vi "SD Module_UI.vi"(8 "error in (no error)":errorcluster, 11 "Node Ptr":T16 format="%.0x") -> (0 "error out":errorcluster)   [LabVIEW 2017, in "Modules.lvlib" / "SD Module.lvclass"]
uses:
  SD Module.lvclass
  Type Defs/_nicrio_TimebaseControl.ctl
  Type Defs/_nicrio_IndexModeControl.ctl
  Type Defs/_nicrio_PeriodControl.ctl
  Type Defs/_nicrio_DriveChanFromCounterControl.ctl
  Type Defs/_nicrio_TerminalCountOutputModeControl.ctl
  Type Defs/_nicrio_GateSourceControl.ctl
  Type Defs/_nicrio_CountEventControl.ctl
  Type Defs/_nicrio_TerminalCountControl.ctl
  Type Defs/_nicrio_CountSourceControl.ctl
  Type Defs/_nicrio_MeasurementModeControl.ctl
  Type Defs/_nicrio_CountDownControl.ctl
  <vilib>/NI Veristand/Custom Device API/Custom Device Item Ref.ctl
  RSI Module/SubPanel Command.ctl
  Type Defs/_nicrio_SpecialtyModeControl.ctl
  Type Defs/_nicrio_InputFilterControl.ctl
  Type Defs/_nicrio_ChannelsControl.ctl
  Type Defs/Quadrature Control Refs.ctl
  Type Defs/Counter Control Refs.ctl
  Type Defs/Main Control Refs.ctl
  Type Defs/SD Control Refs.ctl
  Type Defs/CDO Control Refs.ctl
  Type Defs/PWM Control Refs.ctl
  RSI Module/Slot Settings.ctl
  RSI Module/Module Models.ctl
  C:/Users/dbuck/Documents/GitHub/Scan-Engine-Custom-Device-Classes/Source/RSI Module/RSI Module.lvclass
  SD Module.lvclass/SD Module.ctl
  RSI Module/Debug.vi
  RSI Module/RSI Module.lvclass
  <resource>/objmgr/cRIO.rc
  Modules.lvlib
  <vilib>/NI Veristand/Custom Device API/Custom Device API.lvlib
panel:
  in  "Channels":T1
  in  "Input Filter":T2=128 items=["1 us"=0, "16 us"=1, "256 us"=2, "4096 us"=3, "Disabled"=128]
  in  "SD Tabs":T3(tab)
  in  "Measurement Type":T4 items=["High Pulse"=3, "Low Pulse"=4, "Most Recent"=5]
  in  "Measurement Edge":T4 items=["Rising Edge", "Falling Edge"]
  in  "Output Mode":T5 caption="Terminal Count Output Mode" items=["Toggle, Reset Off", "Toggle, Reset On", "On Pulse", "Off Pulse"]
  in  "Gate Mode":T6 items=["Always Enabled"=3, "Next Channel"=1]
  in  "Counter Event":T4 items=["Rising Edge", "Falling Edge", "Any Edge"]
  in  "Terminal Count":T7=4294967296 min=1 max=4294967296
  in  "Counter Source":T8 items=["This Channel", "Terminal Count of Previous Channel"]
  in  "Frequency Timebase":T9 items=["256 us", "512 us", "1024 us", "2048 us", "4096 us", "8192 us", "16384 us", "32768 us"]
  in  "Measurement Mode":T10 items=["Count Edges", "Period Measurement", "Pulse Width Measurement", "Frequency Measurement"]
  in  "Count Direction":T11 items=["Count Up", "Count Down"]
  in  "Channel Mode":T12 caption="Counter Driven" items=["Disabled", "Enabled"]
  in  "Drive From Slot":u16(ring) items=["Slot 1", "Slot 2", "Slot 3", "Slot 4", "Slot 5", "Slot 6", "Slot 7", "Slot 8"]
  in  "Frequency (Period)":T13=4 items=["1 Hz (1,000,000 us)", "50 Hz (20,000 us)", "250 Hz (4,000 us)", "500 Hz (2,000 us)", "1 kHz (1,000 us)", "5 kHz (200 us)", "10 kHz (100 us)", "20 kHz (50 us)"]
  in  "Velocity Timebase":T9 items=["256 us", "512 us", "1024 us", "2048 us", "4096 us", "8192 us", "16384 us", "32768 us"]
  in  "Index Mode":T14 items=["Disabled", "Phase B0 A0", "Phase B0 A1", "Phase B1 A0", "Phase B1 A1"]
  in  "Specialty Mode":T15 items=["None", "Counter", "Counter-Driven Output", "Pulse-Width Modulation", "Quadrature"]
  in  "SubPanel Event":refnum<user-event>
  in  "Header":cluster{"Section Name":string}={"Section Name"="NI 9205 Settings"}
  # "When in quadrature mode, the A, B, and index channels are the first, second, and third input lines respectively. Modules with six or more digital inputs use successive blocks of three channels to instantiate additional quadratures in the same pattern."
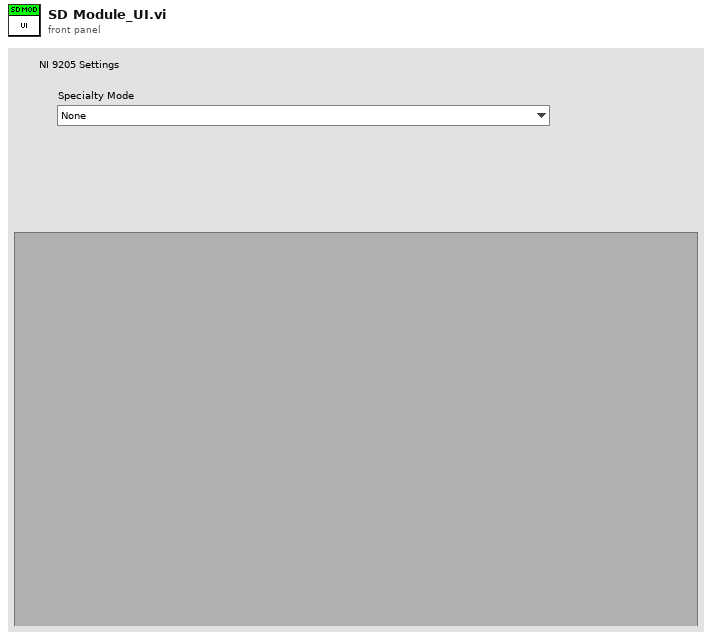
[diagram p1: front panel]
types:
  T1 = typedef "Modules.lvlib/SD Module.lvclass/_nicrio_ChannelsControl.ctl" = i32
  T2 = typedef "Modules.lvlib/SD Module.lvclass/_nicrio_InputFilterControl.ctl" = u16
  T3 = enum32{"Normal", "Counter", "Counter Output", "PWM", "Quadrature", "Error"}
  T4 = typedef "Modules.lvlib/SD Module.lvclass/_nicrio_CountEventControl.ctl" = u16
  T5 = typedef "Modules.lvlib/SD Module.lvclass/_nicrio_TerminalCountOutputModeControl.ctl" = u16
  T6 = typedef "Modules.lvlib/SD Module.lvclass/_nicrio_GateSourceControl.ctl" = u16
  T7 = typedef "Modules.lvlib/SD Module.lvclass/_nicrio_TerminalCountControl.ctl" = u64
  T8 = typedef "Modules.lvlib/SD Module.lvclass/_nicrio_CountSourceControl.ctl" = u16
  T9 = typedef "Modules.lvlib/SD Module.lvclass/_nicrio_TimebaseControl.ctl" = u16
  T10 = typedef "Modules.lvlib/SD Module.lvclass/_nicrio_MeasurementModeControl.ctl" = u16
  T11 = typedef "Modules.lvlib/SD Module.lvclass/_nicrio_CountDownControl.ctl" = u16
  T12 = typedef "Modules.lvlib/SD Module.lvclass/_nicrio_DriveChanFromCounterControl.ctl" = u16
  T13 = typedef "Modules.lvlib/SD Module.lvclass/_nicrio_PeriodControl.ctl" = u16
  T14 = typedef "Modules.lvlib/SD Module.lvclass/_nicrio_IndexModeControl.ctl" = u16
  T15 = typedef "Modules.lvlib/SD Module.lvclass/_nicrio_SpecialtyModeControl.ctl" = u16
  T16 = typedef "Custom Device API.lvlib/Custom Device Item Ref.ctl" = u64
  T17 = typedef "Modules.lvlib/SD Module.lvclass/PWM Control Refs.ctl" = cluster{"Frequency (Period)":refnum<vi>}
  T18 = typedef "Modules.lvlib/SD Module.lvclass/CDO Control Refs.ctl" = cluster{"Drive From Slot":refnum<vi>, "Channel Mode":refnum<vi>}
  T19 = typedef "Modules.lvlib/SD Module.lvclass/SD Control Refs.ctl" = cluster{"Main Control Refs":T20, "Counter Control Refs":T21, "CDO Control Refs":T18, "PWM Control Refs":T17, "Quadrature Control Refs":T22}
  T20 = typedef "Modules.lvlib/SD Module.lvclass/Main Control Refs.ctl" = cluster{"Specialty Mode":refnum<vi>, "Input Filter":refnum<vi>, "SD Tabs":refnum<vi>, "Channels":refnum<vi>, "Non-SD Subpanel":refnum<vi>}
  T21 = typedef "Modules.lvlib/SD Module.lvclass/Counter Control Refs.ctl" = cluster{"Measurement Mode":refnum<vi>, "Counter Event":refnum<vi>, "Counter Source":refnum<vi>, "Count Direction":refnum<vi>, "Terminal Count":refnum<vi>, "Output Mode":refnum<vi>, "Gate Mode":refnum<vi>, "Measurement Edge":refnum<vi>, "Measurement Type":refnum<vi>, "Frequency Timebase":refnum<vi>}
  T22 = typedef "Modules.lvlib/SD Module.lvclass/Quadrature Control Refs.ctl" = cluster{"Velocity Timebase":refnum<vi>, "Index Mode":refnum<vi>}
  T23 = typedef "Modules.lvlib/RSI Module.lvclass/Module Models.ctl" = enum16{"Empty", "NI 9201", "NI 9203", "NI 9205", "NI 9206", "NI 9207", "NI 9208", "NI 9211", "NI 9212", "NI 9213", "NI 9214", "NI 9215", "NI 9217", "NI 9219", "NI 9220", "NI 9221", "NI 9222", "NI 9223", "NI 9225", "NI 9227", "NI 9229", "NI 9233", "NI 9234", "NI 9235", "NI 9236", "NI 9237", "NI 9239", "NI 9242", "NI 9244", "NI 9263", "NI 9264", "NI 9265", "NI 9269", "NI 9375", "NI 9401", "NI 9402", "NI 9403", "NI 9411", "NI 9421", "NI 9422", "NI 9423", "NI 9425", "NI 9426", "NI 9435", "NI 9437", "NI 9472", "NI 9474", "NI 9475", "NI 9476", "NI 9477", "NI 9478", "NI 9481", "NI 9482", "NI 9485"}
  T24 = typedef "Modules.lvlib/RSI Module.lvclass/Slot Settings.ctl" = cluster{"Slot":u32, "EtherCAT?":bool}
  T25 = typedef "Modules.lvlib/RSI Module.lvclass/SubPanel Command.ctl" = enum16{"Stop"}
  T26 = typedef "Modules.lvlib/SD Module.lvclass/CDO Channel.ctl" = cluster{"Counter driven enabled":bool}
  T27 = typedef "Modules.lvlib/SD Module.lvclass/Quadrature Channel.ctl" = cluster{"Timebase":u32, "Index Mode":u32}
  T28 = typedef "Modules.lvlib/SD Module.lvclass/Counter Channel.ctl" = cluster{"Measurement Mode":u32, "Count Edges":T29, "Period Measurement":T30, "Pulse Width Measurement":T31, "Frequency Measurement":T32}
  T29 = typedef "Modules.lvlib/SD Module.lvclass/Count Edges.ctl" = cluster{"Counter Event":u32, "Counter Source":u32, "Counter Direction":u32, "Terminal Count":u32, "Output Mode":u32, "Gate Mode":u32}
  T30 = typedef "Modules.lvlib/SD Module.lvclass/Period Measurement.ctl" = cluster{"Measurement Edge":u32}
  T31 = typedef "Modules.lvlib/SD Module.lvclass/Pulse Width Measurement.ctl" = cluster{"Measurement Type":u32}
  T32 = typedef "Modules.lvlib/SD Module.lvclass/Frequency Measurement.ctl" = cluster{"Measurement Edge":u32, "Measurement Timebase":u32}
  T33 = typedef "Modules.lvlib/SD Module.lvclass/PWM Channel.ctl" = cluster{"PWM frequency":u32}
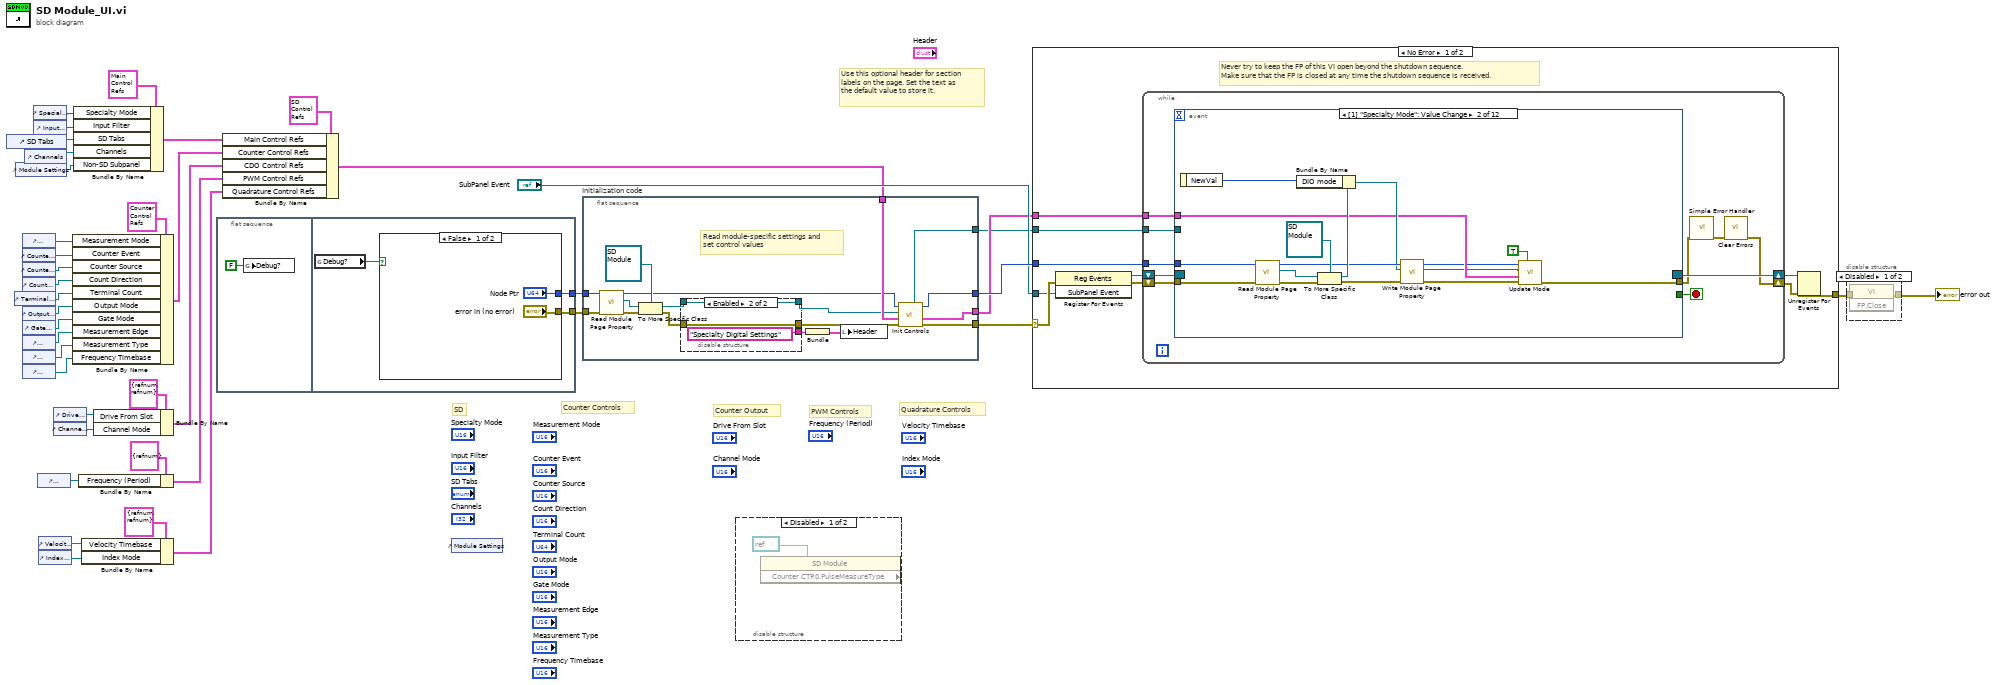
[diagram p0: block diagram]
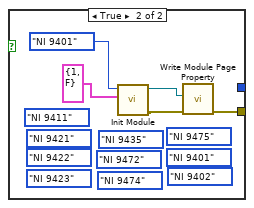
[diagram p3: hidden frame]
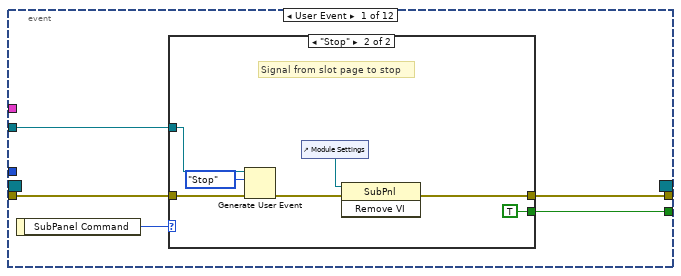
[diagram p4: hidden frame]
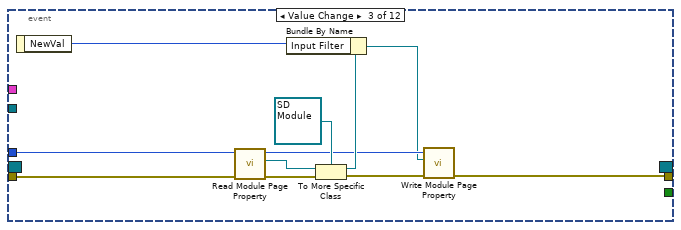
[diagram p6: hidden frame]
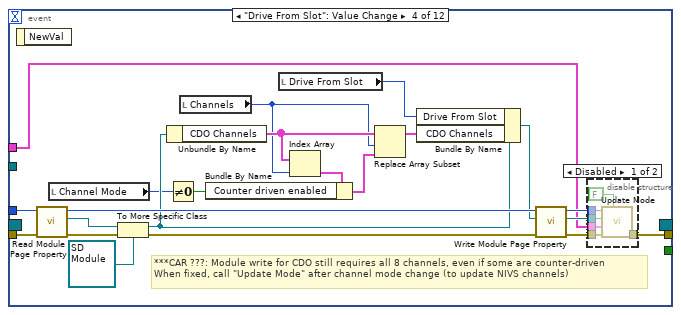
[diagram p7: hidden frame]
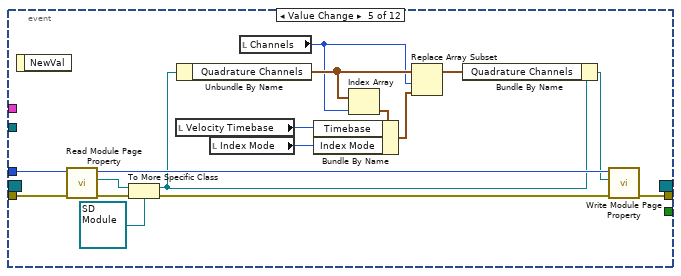
[diagram p9: hidden frame]
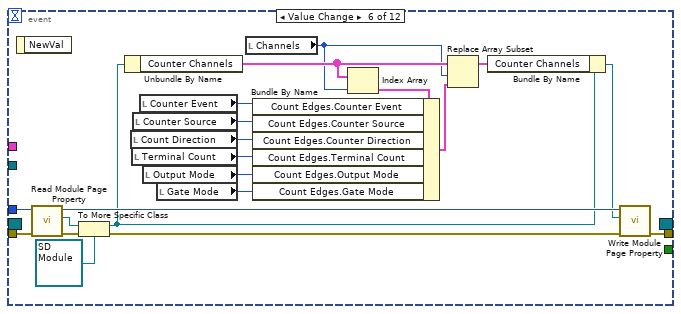
[diagram p10: hidden frame]
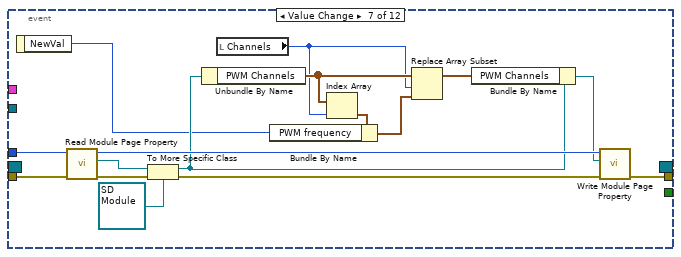
[diagram p11: hidden frame]
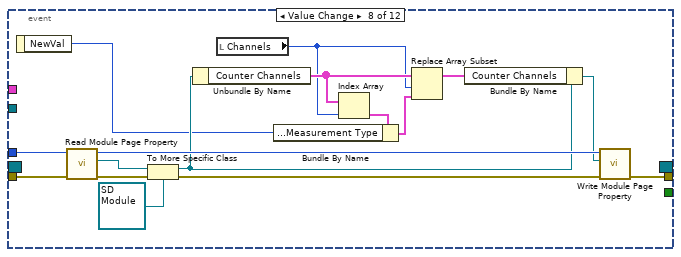
[diagram p12: hidden frame]
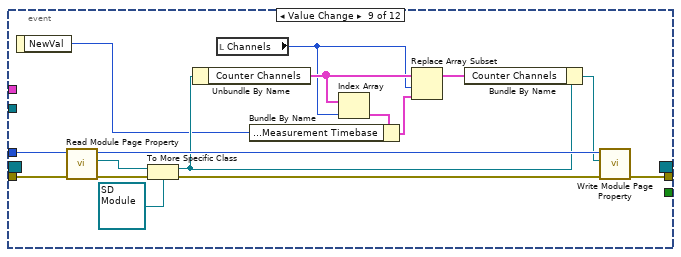
[diagram p13: hidden frame]
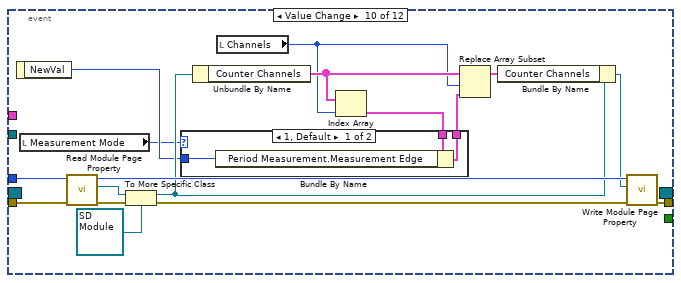
[diagram p14: hidden frame]
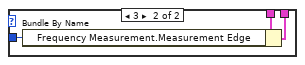
[diagram p15: hidden frame]
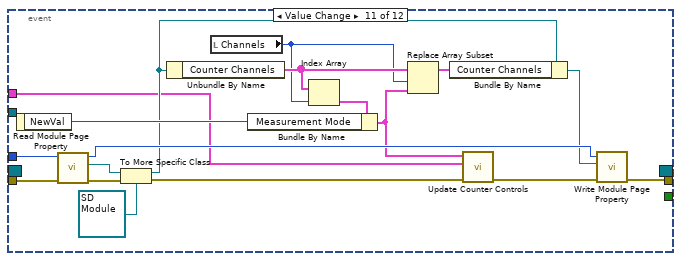
[diagram p16: hidden frame]
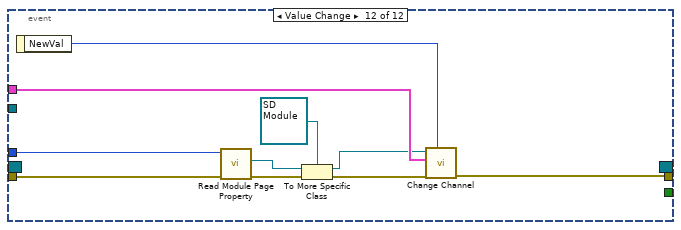
[diagram p17: hidden frame]
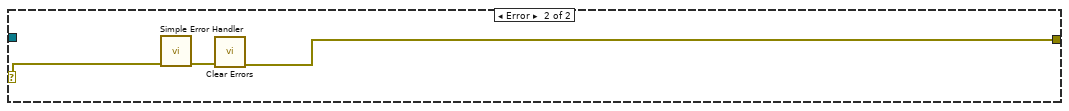
[diagram p18: hidden frame]
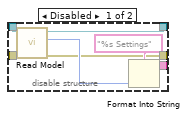
[diagram p19: hidden frame]
diagram:
  # "Counter Output"
  # "Quadrature Controls"
  # "Counter Controls"
  # "PWM Controls"
  # "SD"
  # "Use this optional header for section labels on the page. Set the text as the default value to store it."
  n1 = control-ref of="SD Tabs"() -> (w16:refnum<vi>)
  n2 = control-ref of="Terminal Count"() -> (w25:refnum<vi>)
  n3 = control-ref of="Module Settings"() -> (w2:refnum<vi>)
  n4 = control-ref of="Measurement Mode"() -> (w29:refnum<vi>)
  n5 = control-ref of="Counter Event"() -> (w28:refnum<vi>)
  n6 = control-ref of="Counter Source"() -> (w27:refnum<vi>)
  n7 = control-ref of="Count Direction"() -> (w26:refnum<vi>)
  n8 = control-ref of="Output Mode"() -> (w24:refnum<vi>)
  n9 = control-ref of="Gate Mode"() -> (w23:refnum<vi>)
  n10 = control-ref of="Measurement Edge"() -> (w22:refnum<vi>)
  n11 = control-ref of="Measurement Type"() -> (w21:refnum<vi>)
  n12 = control-ref of="Frequency Timebase"() -> (w20:refnum<vi>)
  n13 = control-ref of="Channels"() -> (w15:refnum<vi>)
  n14 = control-ref of="Specialty Mode"() -> (w18:refnum<vi>)
  n15 = control-ref of="Input Filter"() -> (w17:refnum<vi>)
  n16 = control-ref of="Frequency (Period)"() -> (w10:refnum<vi>)
  n17 = control-ref of="Velocity Timebase"() -> (w40:refnum<vi>)
  n18 = control-ref of="Index Mode"() -> (w39:refnum<vi>)
  n19 = control-ref of="Drive From Slot"() -> (w13:refnum<vi>)
  n20 = control-ref of="Channel Mode"() -> (w12:refnum<vi>)
  n21 = Bundle By Name(cluster=T21 {"Measurement Mode"=refnum, "Counter Event"=refnum, "Counter Source"=refnum, "Count Direction"=refnum, "Terminal Count"=refnum, "Output Mode"=refnum, "Gate Mode"=refnum, "Measurement Edge"=refnum, "Measurement Type"=refnum, "Frequency Timebase"=refnum} ("Counter Control Refs"), "Measurement Mode"=w29, "Counter Event"=w28, "Counter Source"=w27, "Count Direction"=w26, "Terminal Count"=w25, "Output Mode"=w24, "Gate Mode"=w23, "Measurement Edge"=w22, "Measurement Type"=w21, "Frequency Timebase"=w20) -> (w7:T21)
  n22 = Bundle By Name(cluster=T20 {"Specialty Mode"=refnum, "Input Filter"=refnum, "SD Tabs"=refnum, "Channels"=refnum, "Non-SD Subpanel"=refnum} ("Main Control Refs"), "Specialty Mode"=w18, "Input Filter"=w17, "SD Tabs"=w16, "Channels"=w15, "Non-SD Subpanel"=w2) -> (w8:T20)
  n23 = Bundle By Name(cluster=T17 {"Frequency (Period)"=refnum} ("PWM Control Refs"), "Frequency (Period)"=w10) -> (w5:T17)
  n24 = Bundle By Name(cluster=T22 {"Velocity Timebase"=refnum, "Index Mode"=refnum} ("Quadrature Control Refs"), "Velocity Timebase"=w40, "Index Mode"=w39) -> (w38:T22)
  n25 = Bundle By Name(cluster=T18 {"Drive From Slot"=refnum, "Channel Mode"=refnum} ("CDO Control Refs"), "Drive From Slot"=w13, "Channel Mode"=w12) -> (w6:T18)
  n26 = flat-sequence {
    tunnel: [w45] -> w36
    tunnel: [w44] -> w35
    frame #0 {
      n27 = global write "Debug.vi" "Debug?"(FALSE ("Debug?")) -> ()
    }
    frame #1 {
      n28 = global read "Debug.vi" "Debug?"() -> (w43:bool)
      n29 = case shown="False" w43 {
        tunnel: ["Node Ptr" _] -> w45
        tunnel: ["error in (no error)" w52] -> w44
        frame False {
        }
        frame True {
          (unwired) Module_Models."NI 9402" ("Module Model")
          (unwired) Module_Models."NI 9401" ("Module Model")
          (unwired) Module_Models."NI 9411" ("Module Model")
          (unwired) Module_Models."NI 9475" ("Module Model")
          (unwired) Module_Models."NI 9474" ("Module Model")
          (unwired) Module_Models."NI 9472" ("Module Model")
          (unwired) Module_Models."NI 9435" ("Module Model")
          (unwired) Module_Models."NI 9423" ("Module Model")
          (unwired) Module_Models."NI 9422" ("Module Model")
          (unwired) Module_Models."NI 9421" ("Module Model")
          n30 = call "Init Module.vi"("Slot Settings"=T24 {"Slot"=1, "EtherCAT?"=FALSE}, "Module Model"=Module_Models."NI 9401") -> ("error out"=w49:errorcluster, "RSI Module out"=w48:refnum<class "RSI Module.lvclass">)  [unwired: 8 in]
          n31 = call "Write Module Page Property.vi"("error in (no error)"=w49, "RSI Module"=w48) -> ("error out"=w52:errorcluster)  [unwired: 7 in, 2 out]
        }
      }
    }
  }
  n32 = Bundle By Name(cluster=T19 {"Main Control Refs"={"Specialty Mode"=refnum, "Input Filter"=refnum, "SD Tabs"=refnum, "Channels"=refnum, "Non-SD Subpanel"=refnum}, "Counter Control Refs"={"Measurement Mode"=refnum, "Counter Event"=refnum, "Counter Source"=refnum, "Count Direction"=refnum, "Terminal Count"=refnum, "Output Mode"=refnum, "Gate Mode"=refnum, "Measurement Edge"=refnum, "Measurement Type"=refnum, "Frequency Timebase"=refnum}, "CDO Control Refs"={"Drive From Slot"=refnum, "Channel Mode"=refnum}, "PWM Control Refs"={"Frequency (Period)"=refnum}, "Quadrature Control Refs"={"Velocity Timebase"=refnum, "Index Mode"=refnum}} ("SD Control Refs"), "Main Control Refs"=w8, "Counter Control Refs"=w7, "CDO Control Refs"=w6, "PWM Control Refs"=w5, "Quadrature Control Refs"=w38) -> (w4:T19)
  n33 = control-ref of="Module Settings"() -> ()  [unwired: 1 out]
  n34 = flat-sequence "Initialization code" {
    tunnel: w35 -> [w68]
    tunnel: w36 -> [w69]
    tunnel: [w59] -> w31
    tunnel: [w55] -> w34
    tunnel: w4 -> [w58]
    tunnel: [w54] -> w3
    tunnel: [w53] -> w1
    frame #0 {
      # "Read module-specific settings and\nset control values"
      n35 = call "Read Module Page Property.vi"("error in (no error)"=w68, "Node Ptr In"=w69) -> ("error out"=w67:errorcluster, "RSI Module"=w66:refnum<class "RSI Module.lvclass">, "Node Ptr Out"=w56:T16)  [unwired: 7 in]
      n36 = To More Specific Class(target class=refnum<class "SD Module.lvclass"> refnum ("Modules.lvlib:SD Module.lvclass"), reference=w66, error in=w67) -> (specific class reference=w65:refnum<class "SD Module.lvclass">, error out=w64:errorcluster)
      n37 = disable-structure shown="Enabled" {
        disable-tunnel: w65 -> [w76 w79]
        disable-tunnel: w64 -> [w75 w78]
        disable-tunnel: [w72 "Specialty Digital Settings" ("format string")] -> w62
        disable-tunnel: [w71 w79] -> w57
        disable-tunnel: [w70 w78] -> w60
        frame Disabled {
          n38 = call "Read Model.vi"("error in (no error)"=w75, "RSI Module in"=w76) -> ("error out"=w70:errorcluster, "Model"=w74:T23, "RSI Module out"=w71:refnum<class "SD Module.lvclass">)  [unwired: 7 in]
          n39 = Format Into String(format string="%s Settings", w74) -> (resulting string=w72:string)  [unwired: 2 in, 1 out]
        }
        frame Enabled {
        }
      }
      n40 = Bundle("format string"=w62) -> (w63:cluster{"format string":string})  [unwired: 1 in]
      n41 = local write "Header"(w63) -> ()
      n42 = call "Init Controls.vi"("error in (no error)"=w60, "SD Control Refs in"=w58, "SD Module in"=w57, "Node Ptr"=w56) -> ("error out"=w59:errorcluster, "SD Control Refs out"=w54:T19, "Node Ptr"=w55:T16, "SubPanel Command"=w53:refnum<user-event>)  [unwired: 3 in, 1 out]
    }
  }
  n43 = disable-structure shown="Disabled" {
    frame Disabled {
      n44 = property class="SD Module" props=["Counter.CTR0.PulseMeasureType"](reference=refnum<k21> refnum ("shared variable refnum in")) -> ()  [unwired: 1 in, 3 out]
    }
    frame Enabled {
    }
  }
  n45 = case shown="No Error" w31 {
    selector: w31 -> [w84 w309]
    tunnel: [w88 w307] -> w37
    tunnel: w34 -> [w85 _]
    tunnel: "SubPanel Event" -> [w83 _]
    tunnel: w3 -> [w82 _]
    tunnel: w1 -> [w81 _]
    frame No Error {
      # "Never try to keep the FP of this VI open beyond the shutdown sequence.\nMake sure that the FP is closed at any time the shutdown sequence is received."
      n46 = register-events(error in=w84, w83) -> (reference out=w86:refnum<event-registration>, error out=w87:errorcluster)  [unwired: 1 in]
      n47 = while {
        tunnel: w85 -> [w96]
        shift-right: [w93] -> w89
        shift-left: w87 -> [w99]
        shift-right: [w100] -> w90
        shift-left: w86 -> [w98]
        tunnel: w82 -> [w92]
        tunnel: w81 -> [w91]
        stop <- w97 stop-if-true
        n48 = event shown="[1] \"Specialty Mode\": Value Change" {
          selector: w98 -> [_ _ _ _ _ _ _ _ _ _ _ _]
          dyn-events: [_ _ _ _ _ _ _ _ _ _ _ _] -> w100
          timeout: _ -> [_ _ _ _ _ _ _ _ _ _ _ _]
          tunnel: w99 -> [w104 w129 w140 w162 w186 w207 w223 w239 w255 w272 w296 w302]
          tunnel: [w103 _ _ _ _ _ _ _ _ _ _ _] -> w97
          tunnel: [w102 w118 w130 w144 w178 w199 w215 w231 w247 w264 w283 w298] -> w95
          tunnel: w96 -> [_ w123 w134 w158 w182 w203 w219 w235 w251 w268 w292 w303]
          tunnel: w92 -> [_ w117 _ w141 _ _ _ _ _ _ w279 w300]
          tunnel: w91 -> [w101 _ _ _ _ _ _ _ _ _ _ _]
          event User Event {
            n49 = event-data() -> ("SubPanel Command"=w105:T25)  [unwired: 1 out]
            n50 = case shown="\"Stop\"" w105 {
              tunnel: w104 -> [w106 w109]
              tunnel: [w106 w108] -> w102
              tunnel: [_ TRUE] -> w103
              tunnel: w101 -> [_ w112]
              frame Default {
              }
              frame "Stop" {
                # "Signal from slot page to stop"
                n51 = Generate User Event(user event=w112, event data cluster=SubPanel_Command."Stop" ("event data"), error in=w109) -> (error out=w110:errorcluster)  [unwired: 1 in, 1 out]
                n52 = control-ref of="Module Settings"() -> (w107:refnum<vi>)
                n53 = invoke class="SubPnl" method="Remove VI"(reference=w107, error in=w110) -> (error out=w108:errorcluster)  [unwired: 1 in, 2 out]
              }
            }
          }
          event Value Change {
            n54 = event-data() -> ("NewVal"=w125:T15)  [unwired: 1 out]
            n55 = call "Read Module Page Property.vi"("error in (no error)"=w129, "Node Ptr In"=w123) -> ("error out"=w127:errorcluster, "RSI Module"=w126:refnum<class "RSI Module.lvclass">, "Node Ptr Out"=w122:T16)  [unwired: 7 in]
            n56 = To More Specific Class(target class=refnum<class "SD Module.lvclass"> refnum ("Modules.lvlib:SD Module.lvclass"), reference=w126, error in=w127) -> (specific class reference=w124:refnum<class "SD Module.lvclass">, error out=w119:errorcluster)
            n57 = Bundle By Name(cluster=w124, "DIO mode"=w125) -> (w121:refnum<class "SD Module.lvclass">)
            n58 = call "Write Module Page Property.vi"("error in (no error)"=w119, "RSI Module"=w121, "Node Ptr In"=w122) -> ("error out"=w120:errorcluster, "RSI Module out"=w116:refnum<class "SD Module.lvclass">, "Node Ptr Out"=w115:T16)  [unwired: 6 in]
            n59 = call "Update Mode.vi"("Go to first chan?"=TRUE, "error in (no error)"=w120, "SD Control Refs in"=w117, "SD Module in"=w116, "Node Ptr In"=w115) -> ("error out"=w118:errorcluster)  [unwired: 3 in, 3 out]
          }
          event Value Change {
            n60 = event-data() -> ("NewVal"=w136:T2)  [unwired: 1 out]
            n61 = call "Read Module Page Property.vi"("error in (no error)"=w140, "Node Ptr In"=w134) -> ("error out"=w138:errorcluster, "RSI Module"=w137:refnum<class "RSI Module.lvclass">, "Node Ptr Out"=w133:T16)  [unwired: 7 in]
            n62 = To More Specific Class(target class=refnum<class "SD Module.lvclass"> refnum ("Modules.lvlib:SD Module.lvclass"), reference=w137, error in=w138) -> (specific class reference=w135:refnum<class "SD Module.lvclass">, error out=w131:errorcluster)
            n63 = Bundle By Name(cluster=w135, "Input Filter"=w136) -> (w132:refnum<class "SD Module.lvclass">)
            n64 = call "Write Module Page Property.vi"("error in (no error)"=w131, "RSI Module"=w132, "Node Ptr In"=w133) -> ("error out"=w130:errorcluster)  [unwired: 6 in, 2 out]
          }
          event "Drive From Slot": Value Change {
            # "***CAR ???: Module write for CDO still requires all 8 channels, even if some are counter-driven\nWhen fixed, call \"Update Mode\" after channel mode change (to update NIVS channels)"
            n65 = event-data() -> ()  [unwired: 2 out]
            n66 = call "Read Module Page Property.vi"("error in (no error)"=w162, "Node Ptr In"=w158) -> ("error out"=w160:errorcluster, "RSI Module"=w159:refnum<class "RSI Module.lvclass">, "Node Ptr Out"=w157:T16)  [unwired: 7 in]
            n67 = local read "Channel Mode"() -> (w148:T12)
            n68 = To More Specific Class(target class=refnum<class "SD Module.lvclass"> refnum ("Modules.lvlib:SD Module.lvclass"), reference=w159, error in=w160) -> (specific class reference=w153:refnum<class "SD Module.lvclass">, error out=w155:errorcluster)
            n69 = Unbundle By Name(w153) -> ("CDO Channels"=w152:T26[])
            n70 = Not Equal To 0?(x=w148) -> (x != 0?=w149:bool)
            n71 = local read "Channels"() -> (w146:T1)
            n72 = local read "Drive From Slot"() -> (w154:u16)
            n73 = Index Array(array=w152, index=w146) -> (element=w150:T26)
            n74 = Bundle By Name(cluster=w150, "Counter driven enabled"=w149) -> (w147:T26)
            n75 = Replace Array Subset(array=w152, new element=w147, index=w146) -> (w151:T26[])
            n76 = Bundle By Name(cluster=w153, "Drive From Slot"=w154, "CDO Channels"=w151) -> (w156:refnum<class "SD Module.lvclass">)
            n77 = call "Write Module Page Property.vi"("error in (no error)"=w155, "RSI Module"=w156, "Node Ptr In"=w157) -> ("error out"=w145:errorcluster, "RSI Module out"=w142:refnum<class "SD Module.lvclass">, "Node Ptr Out"=w143:T16)  [unwired: 6 in]
            n78 = disable-structure shown="Disabled" {
              disable-tunnel: w145 -> [w168 w169]
              disable-tunnel: [w167 w169] -> w144
              disable-tunnel: w143 -> [w166 _]
              disable-tunnel: w142 -> [w165 _]
              disable-tunnel: w141 -> [w164 _]
              frame Disabled {
                n79 = call "Update Mode.vi"("Go to first chan?"=FALSE, "error in (no error)"=w168, "SD Control Refs in"=w164, "SD Module in"=w165, "Node Ptr In"=w166) -> ("error out"=w167:errorcluster)  [unwired: 3 in, 3 out]
              }
              frame Enabled {
              }
            }
          }
          event Value Change {
            n80 = event-data() -> ()  [unwired: 2 out]
            n81 = call "Read Module Page Property.vi"("error in (no error)"=w186, "Node Ptr In"=w182) -> ("error out"=w184:errorcluster, "RSI Module"=w183:refnum<class "RSI Module.lvclass">, "Node Ptr Out"=w181:T16)  [unwired: 7 in]
            n82 = To More Specific Class(target class=refnum<class "SD Module.lvclass"> refnum ("Modules.lvlib:SD Module.lvclass"), reference=w183, error in=w184) -> (specific class reference=w177:refnum<class "SD Module.lvclass">, error out=w179:errorcluster)
            n83 = local read "Velocity Timebase"() -> (w170:T9)
            n84 = Unbundle By Name(w177) -> ("Quadrature Channels"=w176:T27[])
            n85 = local read "Index Mode"() -> (w171:T14)
            n86 = local read "Channels"() -> (w172:T1)
            n87 = Index Array(array=w176, index=w172) -> (element=w174:T27)
            n88 = Bundle By Name(cluster=w174, "Timebase"=w170, "Index Mode"=w171) -> (w173:T27)
            n89 = Replace Array Subset(array=w176, new element=w173, index=w172) -> (w175:T27[])
            n90 = Bundle By Name(cluster=w177, "Quadrature Channels"=w175) -> (w180:refnum<class "SD Module.lvclass">)
            n91 = call "Write Module Page Property.vi"("error in (no error)"=w179, "RSI Module"=w180, "Node Ptr In"=w181) -> ("error out"=w178:errorcluster)  [unwired: 6 in, 2 out]
          }
          event Value Change {
            n92 = event-data() -> ()  [unwired: 2 out]
            n93 = call "Read Module Page Property.vi"("error in (no error)"=w207, "Node Ptr In"=w203) -> ("error out"=w205:errorcluster, "RSI Module"=w204:refnum<class "RSI Module.lvclass">, "Node Ptr Out"=w202:T16)  [unwired: 7 in]
            n94 = To More Specific Class(target class=refnum<class "SD Module.lvclass"> refnum ("Modules.lvlib:SD Module.lvclass"), reference=w204, error in=w205) -> (specific class reference=w198:refnum<class "SD Module.lvclass">, error out=w200:errorcluster)
            n95 = Unbundle By Name(w198) -> ("Counter Channels"=w197:T28[])
            n96 = local read "Count Direction"() -> (w190:T11)
            n97 = local read "Terminal Count"() -> (w189:T7)
            n98 = local read "Counter Source"() -> (w191:T8)
            n99 = local read "Counter Event"() -> (w192:T4)
            n100 = local read "Output Mode"() -> (w188:T5)
            n101 = local read "Gate Mode"() -> (w187:T6)
            n102 = local read "Channels"() -> (w193:T1)
            n103 = Index Array(array=w197, index=w193) -> (element=w195:T28)
            n104 = Bundle By Name(cluster=w195, "Count Edges.Counter Event"=w192, "Count Edges.Counter Source"=w191, "Count Edges.Counter Direction"=w190, "Count Edges.Terminal Count"=w189, "Count Edges.Output Mode"=w188, "Count Edges.Gate Mode"=w187) -> (w194:T28)
            n105 = Replace Array Subset(array=w197, new element=w194, index=w193) -> (w196:T28[])
            n106 = Bundle By Name(cluster=w198, "Counter Channels"=w196) -> (w201:refnum<class "SD Module.lvclass">)
            n107 = call "Write Module Page Property.vi"("error in (no error)"=w200, "RSI Module"=w201, "Node Ptr In"=w202) -> ("error out"=w199:errorcluster)  [unwired: 6 in, 2 out]
          }
          event Value Change {
            n108 = event-data() -> ("NewVal"=w208:T13)  [unwired: 1 out]
            n109 = call "Read Module Page Property.vi"("error in (no error)"=w223, "Node Ptr In"=w219) -> ("error out"=w221:errorcluster, "RSI Module"=w220:refnum<class "RSI Module.lvclass">, "Node Ptr Out"=w218:T16)  [unwired: 7 in]
            n110 = To More Specific Class(target class=refnum<class "SD Module.lvclass"> refnum ("Modules.lvlib:SD Module.lvclass"), reference=w220, error in=w221) -> (specific class reference=w214:refnum<class "SD Module.lvclass">, error out=w216:errorcluster)
            n111 = Unbundle By Name(w214) -> ("PWM Channels"=w213:T33[])
            n112 = local read "Channels"() -> (w209:T1)
            n113 = Index Array(array=w213, index=w209) -> (element=w211:T33)
            n114 = Bundle By Name(cluster=w211, "PWM frequency"=w208) -> (w210:T33)
            n115 = Replace Array Subset(array=w213, new element=w210, index=w209) -> (w212:T33[])
            n116 = Bundle By Name(cluster=w214, "PWM Channels"=w212) -> (w217:refnum<class "SD Module.lvclass">)
            n117 = call "Write Module Page Property.vi"("error in (no error)"=w216, "RSI Module"=w217, "Node Ptr In"=w218) -> ("error out"=w215:errorcluster)  [unwired: 6 in, 2 out]
          }
          event Value Change {
            n118 = event-data() -> ("NewVal"=w224:T4)  [unwired: 1 out]
            n119 = call "Read Module Page Property.vi"("error in (no error)"=w239, "Node Ptr In"=w235) -> ("error out"=w237:errorcluster, "RSI Module"=w236:refnum<class "RSI Module.lvclass">, "Node Ptr Out"=w234:T16)  [unwired: 7 in]
            n120 = To More Specific Class(target class=refnum<class "SD Module.lvclass"> refnum ("Modules.lvlib:SD Module.lvclass"), reference=w236, error in=w237) -> (specific class reference=w230:refnum<class "SD Module.lvclass">, error out=w232:errorcluster)
            n121 = Unbundle By Name(w230) -> ("Counter Channels"=w229:T28[])
            n122 = local read "Channels"() -> (w225:T1)
            n123 = Index Array(array=w229, index=w225) -> (element=w227:T28)
            n124 = Bundle By Name(cluster=w227, "Pulse Width Measurement.Measurement Type"=w224) -> (w226:T28)
            n125 = Replace Array Subset(array=w229, new element=w226, index=w225) -> (w228:T28[])
            n126 = Bundle By Name(cluster=w230, "Counter Channels"=w228) -> (w233:refnum<class "SD Module.lvclass">)
            n127 = call "Write Module Page Property.vi"("error in (no error)"=w232, "RSI Module"=w233, "Node Ptr In"=w234) -> ("error out"=w231:errorcluster)  [unwired: 6 in, 2 out]
          }
          event Value Change {
            n128 = event-data() -> ("NewVal"=w240:T9)  [unwired: 1 out]
            n129 = call "Read Module Page Property.vi"("error in (no error)"=w255, "Node Ptr In"=w251) -> ("error out"=w253:errorcluster, "RSI Module"=w252:refnum<class "RSI Module.lvclass">, "Node Ptr Out"=w250:T16)  [unwired: 7 in]
            n130 = To More Specific Class(target class=refnum<class "SD Module.lvclass"> refnum ("Modules.lvlib:SD Module.lvclass"), reference=w252, error in=w253) -> (specific class reference=w246:refnum<class "SD Module.lvclass">, error out=w248:errorcluster)
            n131 = Unbundle By Name(w246) -> ("Counter Channels"=w245:T28[])
            n132 = local read "Channels"() -> (w241:T1)
            n133 = Index Array(array=w245, index=w241) -> (element=w243:T28)
            n134 = Bundle By Name(cluster=w243, "Frequency Measurement.Measurement Timebase"=w240) -> (w242:T28)
            n135 = Replace Array Subset(array=w245, new element=w242, index=w241) -> (w244:T28[])
            n136 = Bundle By Name(cluster=w246, "Counter Channels"=w244) -> (w249:refnum<class "SD Module.lvclass">)
            n137 = call "Write Module Page Property.vi"("error in (no error)"=w248, "RSI Module"=w249, "Node Ptr In"=w250) -> ("error out"=w247:errorcluster)  [unwired: 6 in, 2 out]
          }
          event Value Change {
            n138 = event-data() -> ("NewVal"=w257:T4)  [unwired: 1 out]
            n139 = local read "Measurement Mode"() -> (w256:T10)
            n140 = call "Read Module Page Property.vi"("error in (no error)"=w272, "Node Ptr In"=w268) -> ("error out"=w270:errorcluster, "RSI Module"=w269:refnum<class "RSI Module.lvclass">, "Node Ptr Out"=w267:T16)  [unwired: 7 in]
            n141 = To More Specific Class(target class=refnum<class "SD Module.lvclass"> refnum ("Modules.lvlib:SD Module.lvclass"), reference=w269, error in=w270) -> (specific class reference=w263:refnum<class "SD Module.lvclass">, error out=w265:errorcluster)
            n142 = Unbundle By Name(w263) -> ("Counter Channels"=w262:T28[])
            n143 = local read "Channels"() -> (w258:T1)
            n144 = Index Array(array=w262, index=w258) -> (element=w260:T28)
            n145 = case shown="1, Default" w256 {
              tunnel: w260 -> [w275 w278]
              tunnel: [w274 w277] -> w259
              tunnel: w257 -> [w273 w276]
              frame 1, Default {
                n146 = Bundle By Name(cluster=w275, "Period Measurement.Measurement Edge"=w273) -> (w274:T28)
              }
              frame 3 {
                n147 = Bundle By Name(cluster=w278, "Frequency Measurement.Measurement Edge"=w276) -> (w277:T28)
              }
            }
            n148 = Replace Array Subset(array=w262, new element=w259, index=w258) -> (w261:T28[])
            n149 = Bundle By Name(cluster=w263, "Counter Channels"=w261) -> (w266:refnum<class "SD Module.lvclass">)
            n150 = call "Write Module Page Property.vi"("error in (no error)"=w265, "RSI Module"=w266, "Node Ptr In"=w267) -> ("error out"=w264:errorcluster)  [unwired: 6 in, 2 out]
          }
          event Value Change {
            n151 = event-data() -> ("NewVal"=w287:T10)  [unwired: 1 out]
            n152 = call "Read Module Page Property.vi"("error in (no error)"=w296, "Node Ptr In"=w292) -> ("error out"=w294:errorcluster, "RSI Module"=w293:refnum<class "RSI Module.lvclass">, "Node Ptr Out"=w291:T16)  [unwired: 7 in]
            n153 = To More Specific Class(target class=refnum<class "SD Module.lvclass"> refnum ("Modules.lvlib:SD Module.lvclass"), reference=w293, error in=w294) -> (specific class reference=w286:refnum<class "SD Module.lvclass">, error out=w281:errorcluster)
            n154 = Unbundle By Name(w286) -> ("Counter Channels"=w290:T28[])
            n155 = local read "Channels"() -> (w289:T1)
            n156 = Index Array(array=w290, index=w289) -> (element=w288:T28)
            n157 = Bundle By Name(cluster=w288, "Measurement Mode"=w287) -> (w282:T28)
            n158 = Replace Array Subset(array=w290, new element=w282, index=w289) -> (w285:T28[])
            n159 = Bundle By Name(cluster=w286, "Counter Channels"=w285) -> (w284:refnum<class "SD Module.lvclass">)
            n160 = call "Update Counter Controls.vi"("error in (no error)"=w281, "SD Control Refs in"=w279, "Counter Channel"=w282) -> ("error out"=w280:errorcluster)  [unwired: 8 in]
            n161 = call "Write Module Page Property.vi"("error in (no error)"=w280, "RSI Module"=w284, "Node Ptr In"=w291) -> ("error out"=w283:errorcluster)  [unwired: 6 in, 2 out]
          }
          event Value Change {
            n162 = event-data() -> ("NewVal"=w297:T1)  [unwired: 1 out]
            n163 = call "Read Module Page Property.vi"("error in (no error)"=w302, "Node Ptr In"=w303) -> ("error out"=w305:errorcluster, "RSI Module"=w304:refnum<class "RSI Module.lvclass">)  [unwired: 7 in, 1 out]
            n164 = To More Specific Class(target class=refnum<class "SD Module.lvclass"> refnum ("Modules.lvlib:SD Module.lvclass"), reference=w304, error in=w305) -> (specific class reference=w299:refnum<class "SD Module.lvclass">, error out=w301:errorcluster)
            n165 = call "Change Channel.vi"("Channel Index"=w297, "error in (no error)"=w301, "SD Control Refs in"=w300, "SD Module in"=w299) -> ("error out"=w298:errorcluster)  [unwired: 5 in, 2 out]
          }
        }
        n166 = call <vilib>:"Simple Error Handler.vi"("error in (no error)"=w95) -> ("error out"=w94:errorcluster)  [unwired: 1 in, 7 out]
        n167 = call <vilib>:"Clear Errors.vi"("error in (no error)"=w94) -> ("error out"=w93:errorcluster)  [unwired: 1 in, 5 out]
      }
      n168 = Unregister For Events(event registration refnum=w90, error in=w89) -> (error out=w88:errorcluster)
    }
    frame Error {
      n169 = call <vilib>:"Simple Error Handler.vi"("error in (no error)"=w309) -> ("error out"=w308:errorcluster)  [unwired: 1 in, 7 out]
      n170 = call <vilib>:"Clear Errors.vi"("error in (no error)"=w308) -> ("error out"=w307:errorcluster)  [unwired: 1 in, 5 out]
    }
  }
  n171 = disable-structure shown="Disabled" {
    disable-tunnel: w37 -> [w311 _]
    disable-tunnel: [w310 _] -> w32
    frame Disabled {
      n172 = invoke class="VI" method="FP.Close"(error in=w311) -> (error out=w310:errorcluster)  [unwired: 2 in, 2 out]
    }
    frame Enabled {
    }
  }
  "error out" <- w32
